vi "connect_objects.vi"(4 "to_object_terminal_index":i32, 5 "from_object_terminal_index":i32, 6 "wait for reply (T)":bool=TRUE, 7 "to_object_reference":i32, 8 "error in":errorcluster, 9 "from_object_reference":i32, 10 "vi_reference":i32) -> (0 "error out":errorcluster, 1 "timed out?":bool, 3 "result":string)   [LabVIEW 2025, in "Scripting Server.lvlib"]
doc: "Connects two terminals of two objects with a wire on the block diagram of a labview vi. To get a new VI use \"new vi\" to add objects to a vi use \"add object\". If a frontpanel control/indicator reference is passed to this function, it will automatically use the corresponding terminal on the block diagram for wiring. Use get_object_terminals before wiring to find out which terminals to wire."
uses:
  Scripting Server.lvlib
  Connect Objects Argument--cluster.ctl
  Connect Objects (Reply Payload)--cluster.ctl
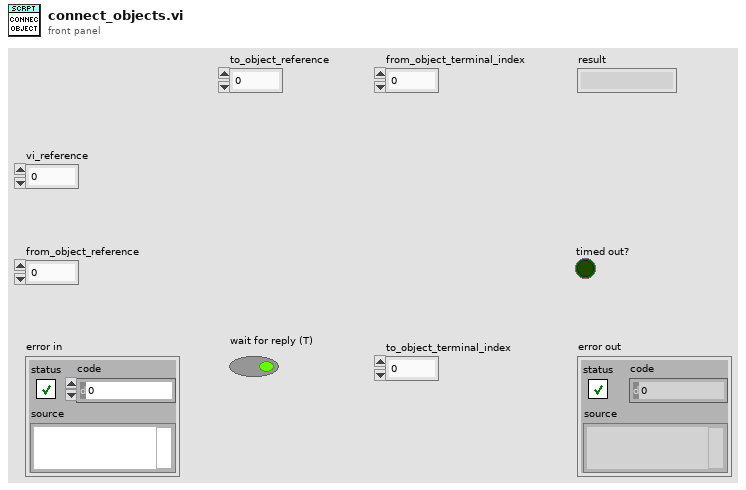
[diagram p1: front panel]
types:
  T1 = typedef "Scripting Server.lvlib/Connect Objects Argument--cluster.ctl" = cluster{"vi reference":i32, "from object reference":i32, "to object reference":i32, "from object terminal index":i32, "to object terminal index":i32, "Wait Notifier":refnum<notifier>, "wait for reply":bool}
  T2 = typedef "Scripting Server.lvlib/Request Events--cluster.ctl" = cluster{"Stop Module":refnum<user-event>, "Show Panel":refnum<user-event>, "Hide Panel":refnum<user-event>, "Get Module Execution Status":refnum<user-event>, "Show Diagram":refnum<user-event>, "New VI":refnum<user-event>, "Add Object":refnum<user-event>, "Connect Objects":refnum<user-event>, "Get Object Terminals":refnum<user-event>, "get vi error list":refnum<user-event>, "Cleanup VI":refnum<user-event>, "create_control":refnum<user-event>, "Run VI":refnum<user-event>, "add_to_selection":refnum<user-event>, "clear_selection_list":refnum<user-event>, "remove_from_selection":refnum<user-event>, "enclose_selection":refnum<user-event>, "rename_object":refnum<user-event>, "set_value":refnum<user-event>, "delete_object":refnum<user-event>, "save_vi":refnum<user-event>, "get_structure_diagram":refnum<user-event>, "add_subvi":refnum<user-event>, "connect_to_pane":refnum<user-event>, "get_object_help":refnum<user-event>, "get_loop_conditional_terminal":refnum<user-event>, "show_conditional_terminal":refnum<user-event>, "get_loop_iteration_terminal":refnum<user-event>, "Read Config Data":refnum<user-event>, "get_allowed_paths":refnum<user-event>, "create_project":refnum<user-event>, "Set Allowed Paths":refnum<user-event>, "open_vi":refnum<user-event>}
  T3 = typedef "Scripting Server.lvlib/Connect Objects (Reply Payload)--cluster.ctl" = cluster{"result":string, "error":errorcluster}
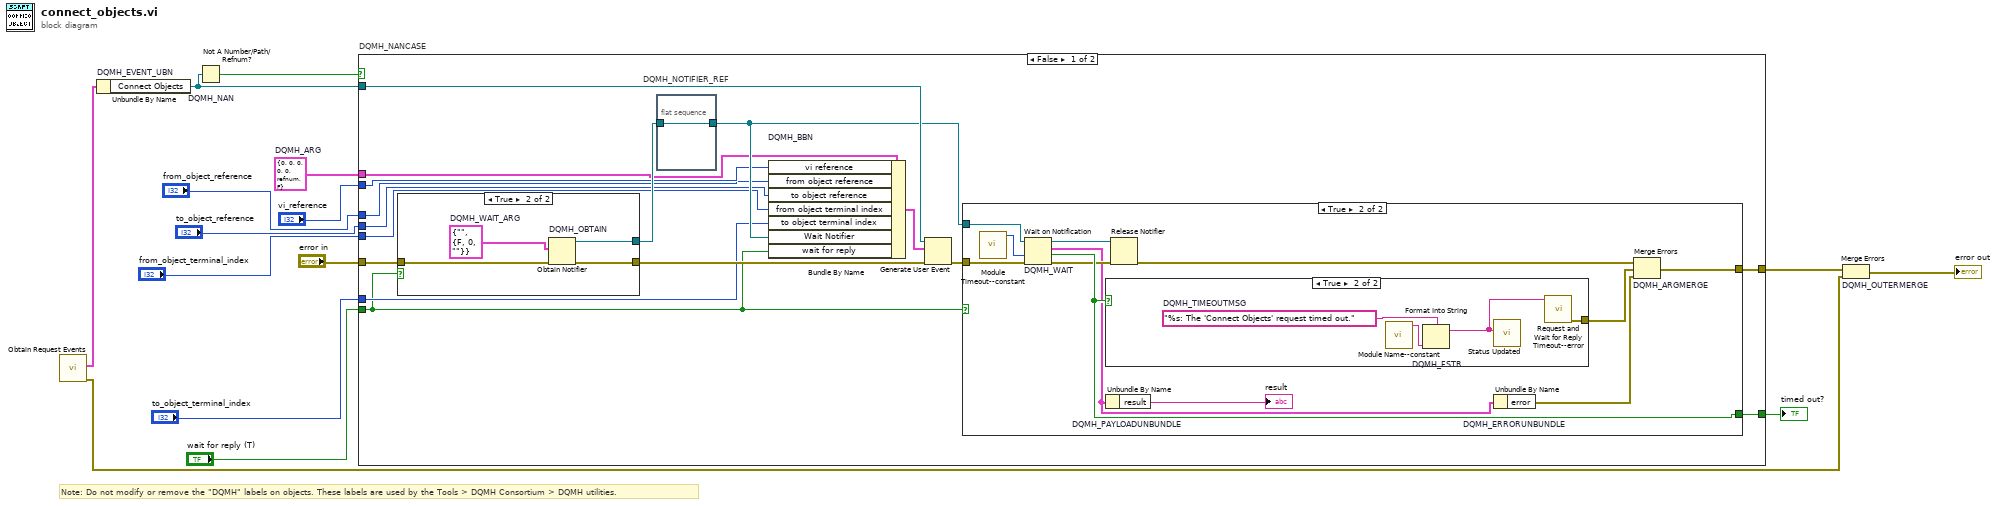
[diagram p0: block diagram]
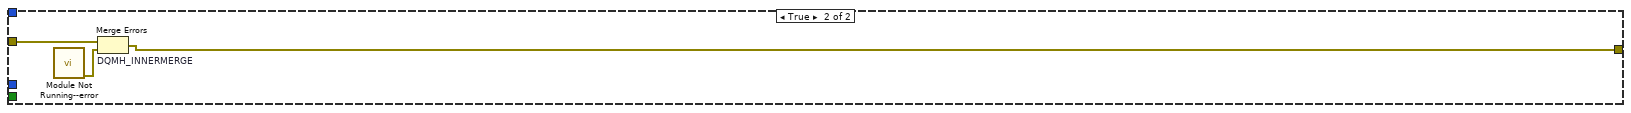
[diagram p5: hidden frame]
diagram:
  w9 = T1 {"vi reference"=0, "from object reference"=0, "to object reference"=0, "from object terminal index"=0, "to object terminal index"=0, "Wait Notifier"=refnum, "wait for reply"=FALSE}  # DQMH_ARG
  # "Note: Do not modify or remove the \"DQMH\" labels on objects. These labels are used by the Tools > DQMH Consortium > DQMH utilities."
  n1 = call "Obtain Request Events.vi"() -> ("error out"=w2:errorcluster, "Scripting Server Request Events"=w1:T2)  [unwired: 10 in]
  n2 = Unbundle By Name "DQMH_EVENT_UBN"(w1) -> ("Connect Objects"=w13:refnum<user-event>)
  n3 = Not A Number/Path/Refnum? "DQMH_NAN"(number/path/refnum=w13) -> (NaN/Path/Refnum?=w12:bool)
  n4 = case "DQMH_NANCASE" shown="False" w12 {
    tunnel: "error in" -> [w31 w57]
    tunnel: w13 -> [w29 _]
    tunnel: [w26 w56] -> w10
    tunnel: [w27 _] -> w11
    tunnel: w9 -> [w22 _]
    tunnel: "vi_reference" -> [w21 _]
    tunnel: "from_object_reference" -> [w20 _]
    tunnel: "to_object_reference" -> [w19 _]
    tunnel: "from_object_terminal_index" -> [w18 _]
    tunnel: "to_object_terminal_index" -> [w17 _]
    tunnel: "wait for reply (T)" -> [w16 _]
    frame False {
      n5 = case shown="True" w16 {
        tunnel: w31 -> [w50 w54]
        tunnel: [w50 w53] -> w28
        tunnel: [_ w51] -> w24
        frame False {
        }
        frame True {
          w52 = T3 {"result"="", "error"={"status"=FALSE, "code"=0, "source"=""}}  # DQMH_WAIT_ARG
          n6 = Obtain Notifier "DQMH_OBTAIN"(notification data type=w52, error in (no error)=w54) -> (notifier out=w51:refnum<notifier>, error out=w53:errorcluster)  [unwired: 2 in, 1 out]
        }
      }
      n7 = flat-sequence "DQMH_NOTIFIER_REF" {
        tunnel: w24 -> [w32]
        tunnel: [w32] -> w23
        frame #0 {
        }
      }
      n8 = Bundle By Name "DQMH_BBN"(cluster=w22, "vi reference"=w21, "from object reference"=w20, "to object reference"=w19, "from object terminal index"=w18, "to object terminal index"=w17, "Wait Notifier"=w23, "wait for reply"=w16) -> (w25:T1)
      n9 = Generate User Event(user event=w29, event data cluster=w25, error in=w28) -> (error out=w30:errorcluster)  [unwired: 1 in, 1 out]
      n10 = case shown="True" w16 {
        tunnel: w30 -> [w33 w45]
        tunnel: w23 -> [_ w44]
        tunnel: [_ w42] -> w27
        tunnel: [w33 w41] -> w26
        frame False {
        }
        frame True {
          n11 = call "Module Timeout--constant.vi"() -> ("Module Timeout"=w35:i32)  [unwired: 11 in]
          n12 = Wait on Notification "DQMH_WAIT"(notifier=w44, timeout in ms (-1)=w35, error in (no error)=w45) -> (notifier out=w43:refnum<notifier>, notification=w36:T3, timed out?=w42:bool, error out=w40:errorcluster)  [unwired: 1 in]
          n13 = case shown="True" w42 {
            tunnel: [_ w47] -> w37
            frame False {
            }
            frame True {
              w49 = "%s: The 'Connect Objects' request timed out."  # DQMH_TIMEOUTMSG
              n14 = call "Module Name--constant.vi"() -> ("Module Name"=w46:string)  [unwired: 11 in]
              n15 = Format Into String "DQMH_FSTR"(format string=w49, w46) -> (resulting string=w48:string)  [unwired: 2 in, 1 out]
              n16 = call "Status Updated.vi"("Status"=w48) -> ()  [unwired: 10 in, 1 out]
              n17 = call "Request and Wait for Reply Timeout--error.vi"("Error Message"=w48) -> ("error out"=w47:errorcluster)  [unwired: 10 in]
            }
          }
          n18 = Unbundle By Name "DQMH_PAYLOADUNBUNDLE"(w36) -> ("result"=→"result":string)
          n19 = Release Notifier(notifier=w43, error in (no error)=w40) -> (error out=w39:errorcluster)  [unwired: 1 in, 2 out]
          n20 = Unbundle By Name "DQMH_ERRORUNBUNDLE"(w36) -> ("error"=w38:errorcluster)
          n21 = Merge Errors "DQMH_ARGMERGE"(w39, w37, w38) -> (w41:errorcluster)
        }
      }
    }
    frame True {
      n22 = call "Module Not Running--error.vi"() -> ("error out"=w55:errorcluster)  [unwired: 11 in]
      n23 = Merge Errors "DQMH_INNERMERGE"(w57, w55) -> (w56:errorcluster)
    }
  }
  "timed out?" <- w11
  n24 = Merge Errors "DQMH_OUTERMERGE"(w10, w2) -> (→"error out":errorcluster)
